vi "myRIO-1900 DaNI FPGA.vi"() -> ()   [LabVIEW 2013]
uses:
  <vilib>/Platform/TimedLoop/XDataNode/timing_clust.ctl
  <vilib>/Platform/TimedLoop/XDataNode/nitl_modes.ctl
  <vilib>/Platform/TimedLoop/XDataNode/wakeup.ctl
  <vilib>/robotics/Utilities/Encoder Count Encoding.ctl
  <vilib>/rvi/Emulation/niFpgaSctlEmulationGetInTimedLoop.vi
  <vilib>/rvi/Emulation/niFpgaProcessEmulError.vi
  <vilib>/rvi/Emulation/niFpgaEmulationReportErrorSimple.vi
  <vilib>/rvi/Emulation/niFpgaGetClockAttributes.vi
  <vilib>/rvi/Emulation/niFpgaCriticalErrorInLSC.vi
  <vilib>/robotics/Starter Kit/2.0/FPGA Source/Globals.vi
  <vilib>/robotics/Utilities/FPGA Utilities/Count Two Phase Digital Encoder.vi
  <vilib>/robotics/Utilities/FPGA Utilities/Generate Digital Pulse (uSec).vi
  <vilib>/Platform/TimedLoop/XDataNode/XDataNode.xnode
  <vilib>/addons/control/pid/fpga.llb/XNode/niFpgaPID.xnode
  <vilib>/Platform/TimedLoop/XDataNode/XDNodeRunTimeDep.lvlib
  <vilib>/robotics/Utilities/NI_Robotics Utilities.lvlib
  <vilib>/robotics/Utilities/FPGA Utilities/NI_Robotics_FPGA Utilities.lvlib
  <vilib>/robotics/Starter Kit/2.0/FPGA Source/NI_Robotics_Starter Kit 2.0 FPGA.lvlib
  <instrlib>/Parallax PING)))/FPGA/NI_Robotics_Parallax PING))) (FPGA).lvlib
  <instrlib>/Hitec HS400 Series/FPGA/NI_Robotics_Hitec HS400 Series (FPGA).lvlib
  <vilib>/robotics/Starter Kit/FPGA Source/NI_Robotics_Starter Kit FPGA.lvlib
panel:
  out "PING)))_0_timeout":bool
  out "PING)))_0_dist":fxp<+,32,8> format="%.27g"
  in  "hs400_0_ccw angle":fxp<+/-,32,4>
  in  "hs400_0_ccw offset":fxp<+/-,32,4>
  in  "servo_0_PWM":T1={"period (us)"=20000, "pulse width (us)"=1500}
  in  "servo_0_direct":bool
  in  "motor PID gains":T2={"proportional gain (Kc)"=0.25, "integral gain (Kc*Ts/Ti)"=0.08984375, "derivative gain (Kc*Td/Ts)"=0.01171875}
  out "DCmotor_0_ccw vel":fxp<+/-,32,11>
  out "DCmotor_1_ccw vel":fxp<+/-,32,11>
  in  "DCmotor_0_direct":bool
  in  "DCmotor_1_direct":bool
  in  "stop":bool
  in  "DCmotor_0_PWM":T1={"period (us)"=20000, "pulse width (us)"=1500}
  in  "DCmotor_1_PWM":T1={"period (us)"=20000, "pulse width (us)"=1500}
  in  "DCmotor_0_ccw vel sp":fxp<+/-,32,11>
  in  "DCmotor_1_ccw vel sp":fxp<+/-,32,11>
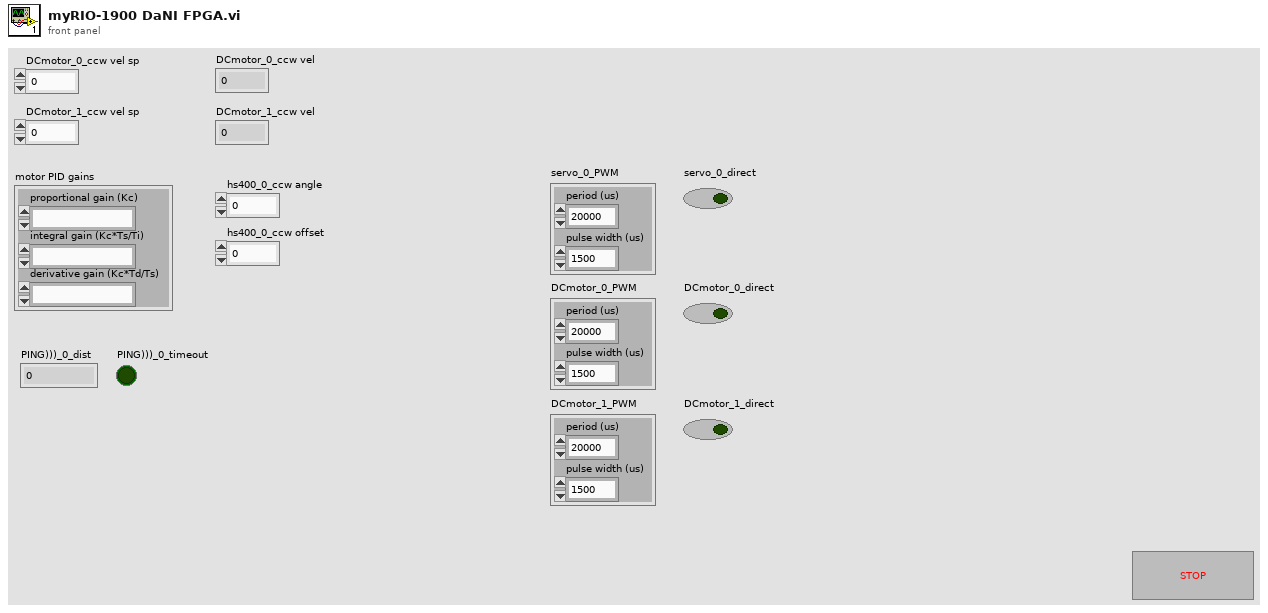
[diagram p1: front panel]
types:
  T1 = cluster{"period (us)":u32, "pulse width (us)":u32}
  T2 = cluster{"proportional gain (Kc)":fxp<+/-,16,8>, "integral gain (Kc*Ts/Ti)":fxp<+/-,16,8>, "derivative gain (Kc*Td/Ts)":fxp<+/-,16,8>}
  T3 = cluster{"PID gains":cluster{"proportional gain (Kc)":fxp<+/-,16,8>, "integral gain (Kc*Ts/Ti)":fxp<+/-,16,8>, "derivative gain (Kc*Td/Ts)":fxp<+/-,16,8>}, "output range":cluster{"output high":fxp<+/-,16,16>, "output low":fxp<+/-,16,16>}, "setpoint":fxp<+/-,16,16>, "channel index":u16}
  T4 = cluster{"PID gains (x 2^8)":cluster{"proportional gain (Kc)":i16, "integral gain (Kc*Ts/Ti)":i16, "derivative gain (Kc*Td/Ts)":i16}, "output range":cluster{"output high":i16, "output low":i16}, "setpoint":i16, "channel index":u16}
  T5 = typedef "XDNodeRunTimeDep.lvlib/timing_clust.ctl" = cluster{"Expected End [f-1]":u64, "Actual End [f-1]":u64, "Finished Late? [f-1]":bool, "Expected End [i-1]":u64, "Actual End [i-1]":u64, "Finished Late? [i-1]":bool, "Expected Start [i]":u64, "Actual Start [i]":u64, "Expected Start [f]":u64, "Actual Start [f]":u64, "Source Name":string, "Structure Name":string, "Period":i64, "Deadline":i64, "Offset":i64, "Start":i64, "Priority":i32, "Timeout":i32, "Mode":T6, "Wakeup Reason":T7, "Error":errorcluster, "Source Type":string, "Secondary Source Type":string, "Global End Time":u64, "Global Start Time":u64, "Frame Duration":u64, "Iteration Duration":u64, "Assigned CPU":i32, "I/O Scan Engine Mode":u32}
  T6 = typedef "XDNodeRunTimeDep.lvlib/nitl_modes.ctl" = enum32{"No Change", "Process missed periods, maintain original phase", "Discard missed periods, maintain original phase", "Process missed periods, ignore original phase", "Discard missed periods, ignore original phase"}
  T7 = typedef "XDNodeRunTimeDep.lvlib/wakeup.ctl" = enum32{"Normal", "Aborted", "Asynchronous wakeup", "Timing source error", "Timed loop error", "Timeout"}
  T8 = typedef "NI_Robotics Utilities.lvlib/Encoder Count Encoding.ctl" = enum16{"X1", "X2", "X4"}
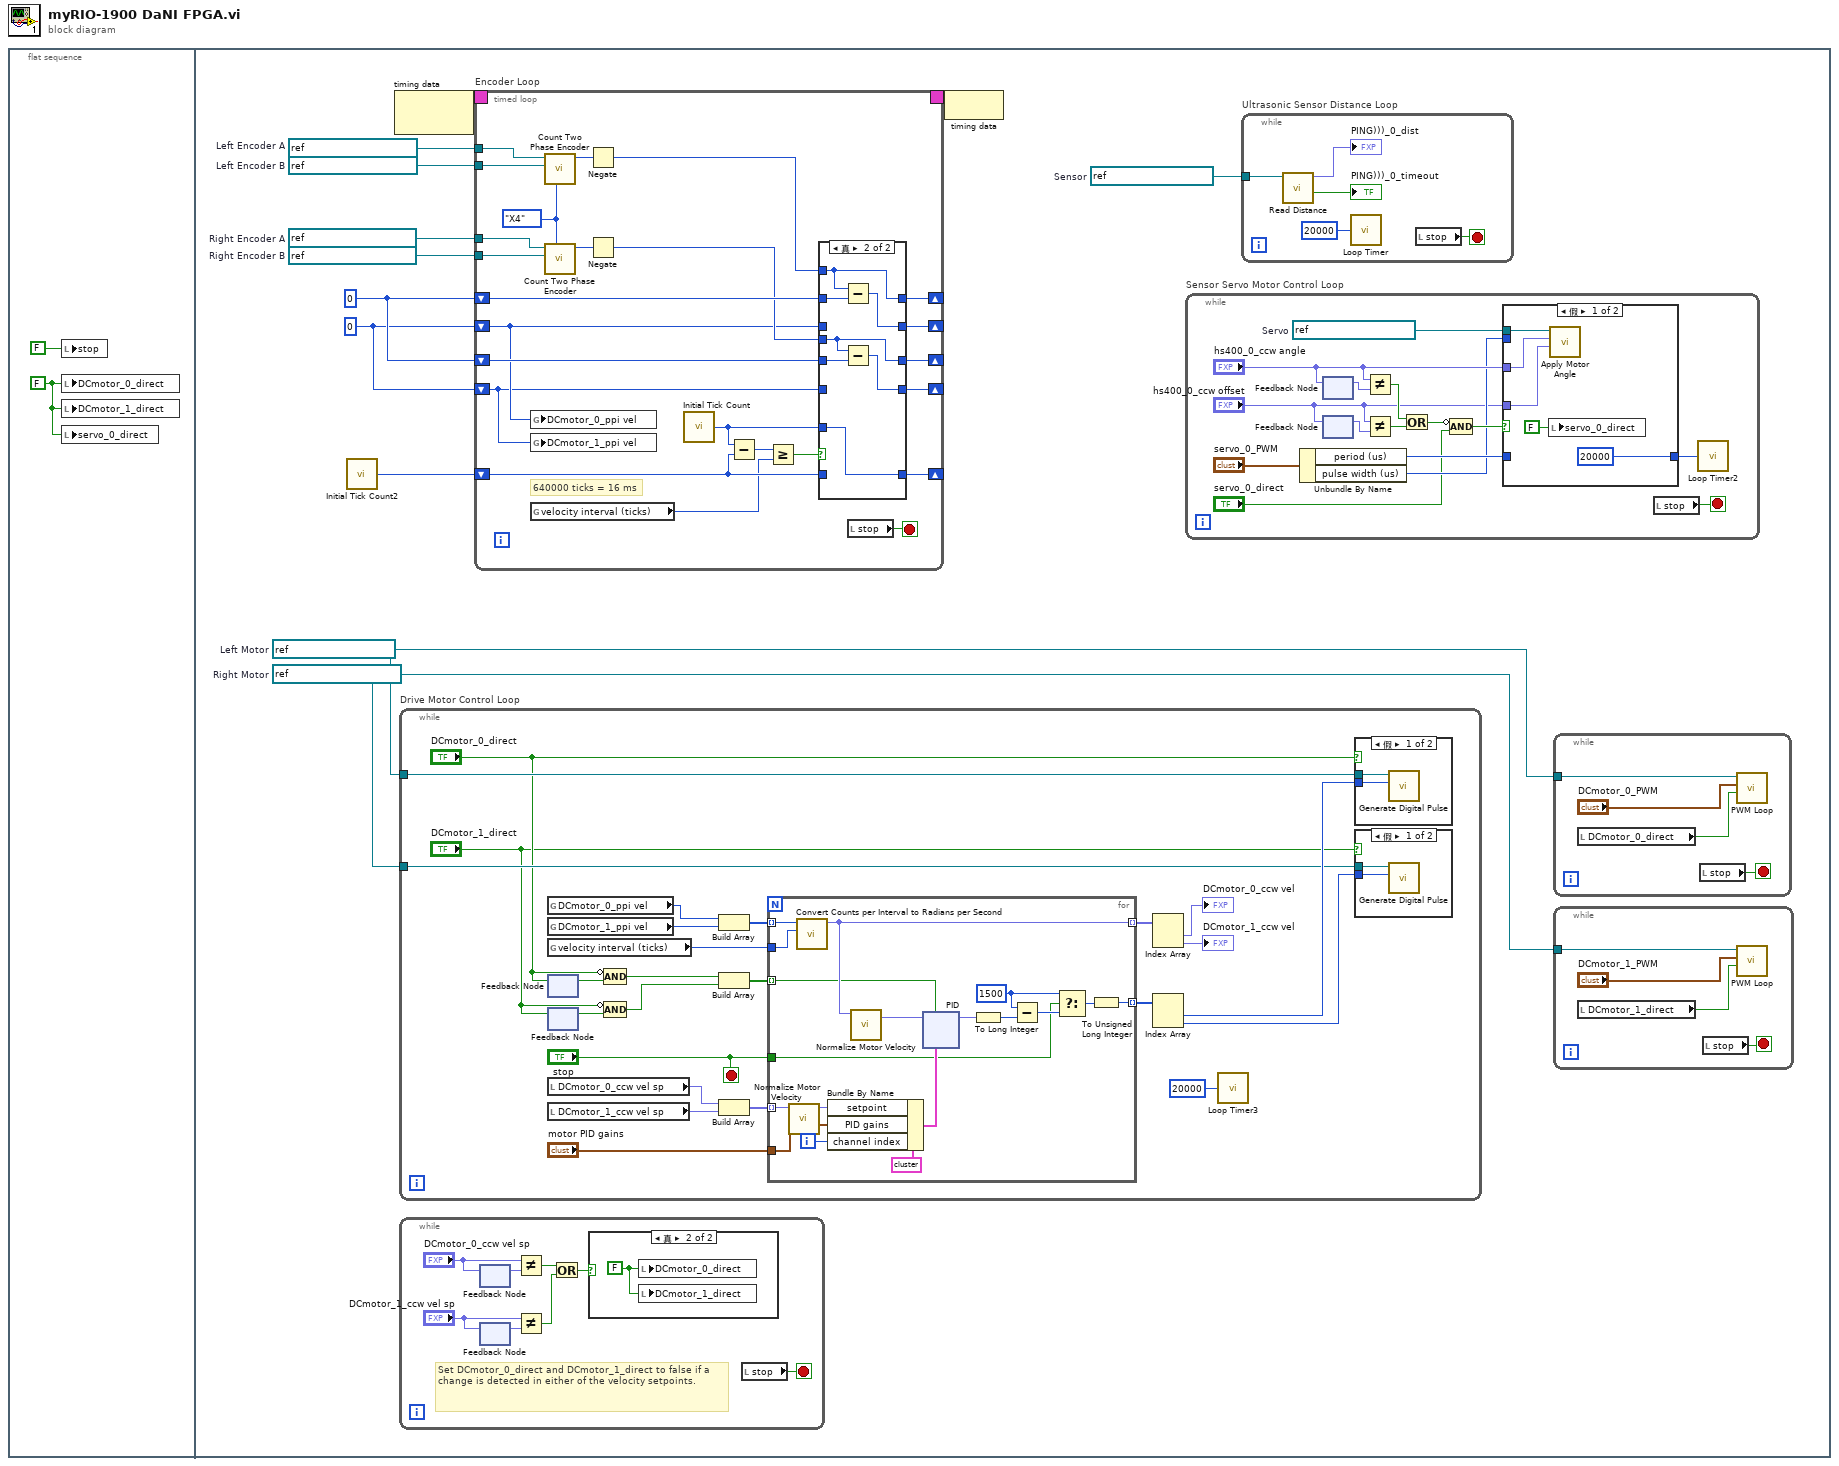
[diagram p0: block diagram]
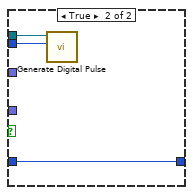
[diagram p5: hidden frame]
diagram:
  n1 = flat-sequence {
    frame #0 {
      w1 = FALSE ("DCmotor_0_direct")
      n2 = local write "stop"(FALSE ("stop")) -> ()
      n3 = local write "DCmotor_0_direct"(w1) -> ()
      n4 = local write "DCmotor_1_direct"(w1) -> ()
      n5 = local write "servo_0_direct"(w1) -> ()
    }
    frame #1 {
      w3 = refnum<k21> "ConnectorA/DIO10"  # Right Motor
      w4 = refnum<k21> "ConnectorA/DIO8"  # Left Motor
      w5 = refnum<k21> "ConnectorB/DIO12"  # Right Encoder B
      w6 = refnum<k21> "ConnectorB/DIO11"  # Right Encoder A
      w7 = refnum<k21> "ConnectorA/DIO12"  # Left Encoder B
      w8 = refnum<k21> "ConnectorA/DIO11"  # Left Encoder A
      w9 = refnum<k21> "ConnectorA/DIO4"  # Sensor
      w10 = 0
      w11 = 0 ("Reset Position Value")
      n6 = call "Initial Tick Count2"() -> ("Tick Count(Ticks)"=w12:u32)
      n7 = node-c288() -> (w14:T5)  [unwired: 1 in]
      n8 = while "Drive Motor Control Loop" {
        tunnel: w4 -> [w49]
        tunnel: w3 -> [w45]
        stop <- "stop" stop-if-true
        n9 = global read "Globals.vi" "DCmotor_0_ppi vel"() -> (w42:i32)
        n10 = global read "Globals.vi" "DCmotor_1_ppi vel"() -> (w41:i32)
        n11 = global read "Globals.vi" "velocity interval (ticks)"() -> (w40:u32)
        n12 = feedback #1() -> (w37:bool)  [unwired: 1 in]
        n13 = feedback-in #1("DCmotor_0_direct") -> ()
        n14 = feedback #2() -> (w38:bool)  [unwired: 1 in]
        n15 = feedback-in #2("DCmotor_1_direct") -> ()
        n16 = local read "DCmotor_0_ccw vel sp"() -> (w44:fxp<+/-,32,11>)
        n17 = local read "DCmotor_1_ccw vel sp"() -> (w43:fxp<+/-,32,11>)
        n18 = Compound Arithmetic op=AND(invert "DCmotor_0_direct", w37) -> (w34:bool)
        n19 = Compound Arithmetic op=AND(invert "DCmotor_1_direct", w38) -> (w33:bool)
        n20 = Build Array(w42, w41) -> (w54:i32[])
        n21 = Build Array(w34, w33) -> (w32:bool[])
        n22 = Build Array(w44, w43) -> (w52:fxp<+/-,32,11>[])
        n23 = for {
          tunnel: "motor PID gains" -> [w75]
          tunnel: w54 -> [w74] mode=indexing
          tunnel: w40 -> [w73]
          tunnel: [w72] -> w53 mode=indexing
          tunnel: w52 -> [w69] mode=indexing
          tunnel: "stop" -> [w62]
          tunnel: [w63] -> w51 mode=indexing
          tunnel: w32 -> [w61] mode=indexing
          i -> [w76]
          w66 = 1500 ("y")
          n24 = call <vilib>:"Normalize Motor Velocity.vi"("velocity (rad/s)"=w69) -> ("normalized velocity"=w70:fxp<+/-,16,16>)  [unwired: 10 in]
          n25 = call <vilib>:"Convert Counts per Interval to Radians per Second.vi"("interval (ticks)"=w73, "velocity (pulses/interval)"=w74) -> ("velocity (rad/s)"=w72:fxp<+/-,32,11>)  [unwired: 9 in]
          n26 = Bundle By Name(cluster=T3 {"PID gains"={"proportional gain (Kc)"=0.00390625, "integral gain (Kc*Ts/Ti)"=0.00390625, "derivative gain (Kc*Td/Ts)"=0.00390625}, "output range"={"output high"=500.0, "output low"=-500.0}, "setpoint"=0.0, "channel index"=0} ("configuration"), "setpoint"=w70, "PID gains"=w75, "channel index"=w76) -> (w77:T3)
          n27 = call <vilib>:"Normalize Motor Velocity.vi"("velocity (rad/s)"=w72) -> ("normalized velocity"=w71:fxp<+/-,16,16>)  [unwired: 10 in]
          n28 = xnode ("PID")("process variable"=w71, "reset?"=w61, "configuration"=w77) -> ("output"=w64:fxp<+/-,16,16>)  [unwired: 1 out]
          n29 = To Long Integer(number=w64) -> (32bit integer=w65:i32)
          n30 = Subtract(x=w66, y=w65) -> (x-y=w67:i32)
          n31 = Select(t=w66, s=w62, f=w67) -> (s? t:f=w68:i32)
          n32 = To Unsigned Long Integer(number=w68) -> (unsigned 32bit integer=w63:u32)
        }
        n33 = Index Array(array=w53) -> (element #1=→"DCmotor_0_ccw vel":fxp<+/-,32,11>, element #2=→"DCmotor_1_ccw vel":fxp<+/-,32,11>)  [unwired: 2 in]
        n34 = Index Array(array=w51) -> (element #1=w50:u32, element #2=w46:u32)  [unwired: 2 in]
        n35 = call "Loop Timer3"("Count(uSec)"=u32 20000) -> ()  [unwired: 1 out]
        n36 = case shown="假" "DCmotor_0_direct" {
          tunnel: w50 -> [w60 _]
          tunnel: w49 -> [w59 _]
          frame False {
            n37 = call-poly <vilib>:"Generate Digital Pulse.vi"("pulse width (uSec)"=w60, "FPGA digital output"=w59) -> ()  [unwired: 10 in]
          }
          frame True {
          }
        }
        n38 = case shown="假" "DCmotor_1_direct" {
          tunnel: w46 -> [w58 _]
          tunnel: w45 -> [w57 _]
          frame False {
            n39 = call-poly <vilib>:"Generate Digital Pulse.vi"("pulse width (uSec)"=w58, "FPGA digital output"=w57) -> ()  [unwired: 10 in]
          }
          frame True {
          }
        }
      }
      n40 = while {
        stop <- w20 stop-if-true
        # "Set DCmotor_0_direct and DCmotor_1_direct to false if a change is detected in either of the velocity setpoints."
        n41 = feedback-in #3("DCmotor_0_ccw vel sp") -> ()
        n42 = feedback #3() -> (w22:fxp<+/-,32,11>)  [unwired: 1 in]
        n43 = feedback #4() -> (w18:fxp<+/-,32,11>)  [unwired: 1 in]
        n44 = feedback-in #4("DCmotor_1_ccw vel sp") -> ()
        n45 = Not Equal?(x="DCmotor_0_ccw vel sp", y=w22) -> (x != y?=w16:bool)
        n46 = Not Equal?(x="DCmotor_1_ccw vel sp", y=w18) -> (x != y?=w17:bool)
        n47 = Or(x=w16, y=w17) -> (x .or. y?=w15:bool)
        n48 = case shown="真" w15 {
          frame False {
          }
          frame True {
            w23 = FALSE ("DCmotor_0_direct")
            n49 = local write "DCmotor_0_direct"(w23) -> ()
            n50 = local write "DCmotor_1_direct"(w23) -> ()
          }
        }
        n51 = local read "stop"() -> (w20:bool)
      }
      n52 = timed-loop "Encoder Loop" {
        timing: w14 -> [_]
        timing-out: [_] -> w13
        shift-right: [w150] -> _
        shift-left: w12 -> [w155]
        shift-right: [w151] -> _
        shift-left: w11 -> [w153]
        shift-right: [w152] -> _
        shift-left: w10 -> [w137]
        shift-right: [w148] -> _
        shift-left: w11 -> [w149]
        shift-right: [w147] -> _
        shift-left: w10 -> [w136]
        tunnel: w8 -> [w144]
        tunnel: w7 -> [w143]
        tunnel: w6 -> [w141]
        tunnel: w5 -> [w140]
        stop <- w134 stop-if-true
        w138 = Encoder_Count_Encoding."X4" ("count multiplier (X1)")
        # "640000 ticks = 16 ms"
        n53 = global write "Globals.vi" "DCmotor_0_ppi vel"(w137) -> ()
        n54 = global write "Globals.vi" "DCmotor_1_ppi vel"(w136) -> ()
        n55 = global read "Globals.vi" "velocity interval (ticks)"() -> (w135:u32)
        n56 = call-poly <vilib>:"Count Two Phase Encoder.vi"("count encoding (X1)"=w138, "phase B FPGA digital input"=w143, "phase A FPGA digital input"=w144) -> ("new count"=w142:i32)  [unwired: 7 in, 1 out]
        n57 = call-poly <vilib>:"Count Two Phase Encoder.vi"("count encoding (X1)"=w138, "phase B FPGA digital input"=w140, "phase A FPGA digital input"=w141) -> ("new count"=w139:i32)  [unwired: 7 in, 1 out]
        n58 = Negate(x=w142) -> (-x=w146:i32)
        n59 = Negate(x=w139) -> (-x=w145:i32)
        n60 = call "Initial Tick Count"() -> ("Tick Count(Ticks)"=w154:u32)
        n61 = Subtract(x=w154, y=w155) -> (x-y=w157:u32)
        n62 = Greater Or Equal?(x=w157, y=w135) -> (x >= y?=w156:bool)
        n63 = case shown="真" w156 {
          tunnel: w154 -> [_ w168]
          tunnel: w155 -> [w162 _]
          tunnel: [w162 w168] -> w150
          tunnel: w153 -> [w161 w169]
          tunnel: [w161 w167] -> w151
          tunnel: w146 -> [_ w167]
          tunnel: [w160 w166] -> w152
          tunnel: w137 -> [w160 _]
          tunnel: w149 -> [w159 w165]
          tunnel: w136 -> [w158 _]
          tunnel: [w159 w164] -> w148
          tunnel: [w158 w163] -> w147
          tunnel: w145 -> [_ w164]
          frame False {
          }
          frame True {
            n64 = Subtract(x=w167, y=w169) -> (x-y=w166:i32)
            n65 = Subtract(x=w164, y=w165) -> (x-y=w163:i32)
          }
        }
        n66 = local read "stop"() -> (w134:bool)
      }
      n67 = node-c288(w13) -> ()
      n68 = while "Sensor Servo Motor Control Loop" {
        stop <- w106 stop-if-true
        w119 = refnum<k21> "ConnectorA/DIO9"  # Servo
        n69 = Unbundle By Name("servo_0_PWM") -> ("period (us)"=w117:u32, "pulse width (us)"=w109:u32)
        n70 = feedback #5() -> (w115:fxp<+/-,32,4>)  [unwired: 1 in]
        n71 = feedback-in #5("hs400_0_ccw angle") -> ()
        n72 = feedback #6() -> (w114:fxp<+/-,32,4>)  [unwired: 1 in]
        n73 = feedback-in #6("hs400_0_ccw offset") -> ()
        n74 = Not Equal?(x="hs400_0_ccw angle", y=w115) -> (x != y?=w112:bool)
        n75 = Not Equal?(x="hs400_0_ccw offset", y=w114) -> (x != y?=w113:bool)
        n76 = Or(x=w112, y=w113) -> (x .or. y?=w111:bool)
        n77 = Compound Arithmetic op=AND(invert w111, "servo_0_direct") -> (w110:bool)
        n78 = case shown="假" w110 {
          tunnel: w109 -> [_ w128]
          tunnel: w119 -> [w123 w127]
          tunnel: "hs400_0_ccw angle" -> [w122 _]
          tunnel: "hs400_0_ccw offset" -> [w121 _]
          tunnel: [u32 20000 ("Count(uSec)") w126] -> w118
          tunnel: w117 -> [_ w126]
          frame False {
            n79 = local write "servo_0_direct"(FALSE ("servo_0_direct")) -> ()
            n80 = call <instrlib>:"Apply Motor Angle.vi"("ccw angle offset (rad)"=w121, "ccw angle (rad)"=w122, "digital output line"=w123) -> ()  [unwired: 9 in]
          }
          frame True {
            n81 = call-poly <vilib>:"Generate Digital Pulse.vi"("pulse width (uSec)"=w128, "FPGA digital output"=w127) -> ()  [unwired: 10 in]
          }
        }
        n82 = local read "stop"() -> (w106:bool)
        n83 = call "Loop Timer2"("Count(uSec)"=w118) -> ()  [unwired: 1 out]
      }
      n84 = while "Ultrasonic Sensor Distance Loop" {
        tunnel: w9 -> [w132]
        stop <- w129 stop-if-true
        n85 = call <instrlib>:"Read Distance.vi"("trigger/echo line"=w132) -> ("timed out?"=→"PING)))_0_timeout":bool, "distance (m)"=→"PING)))_0_dist":fxp<+,32,8>)  [unwired: 9 in]
        n86 = call "Loop Timer"("Count(uSec)"=u32 20000 ("sensor period (15000 us)")) -> ()  [unwired: 1 out]
        n87 = local read "stop"() -> (w129:bool)
      }
      n88 = while {
        tunnel: w4 -> [w30]
        stop <- w28 stop-if-true
        n89 = local read "DCmotor_0_direct"() -> (w29:bool)
        n90 = local read "stop"() -> (w28:bool)
        n91 = call <vilib>:"PWM Loop.vi"("generate pulse (T)"=w29, "PWM"="DCmotor_0_PWM", "FPGA I/O"=w30) -> ()  [unwired: 9 in]
      }
      n92 = while {
        tunnel: w3 -> [w27]
        stop <- w24 stop-if-true
        n93 = local read "DCmotor_1_direct"() -> (w25:bool)
        n94 = local read "stop"() -> (w24:bool)
        n95 = call <vilib>:"PWM Loop.vi"("generate pulse (T)"=w25, "PWM"="DCmotor_1_PWM", "FPGA I/O"=w27) -> ()  [unwired: 9 in]
      }
    }
  }
